vi "ClsDownloadDeviceSpectrumSingleChannelDevice.vi"(8 "error in":errorcluster, 10 "Spectrum Type":i32, 11 "Connection In":u32) -> (0 "error out":errorcluster, 2 "Spectrum":i16[](array[numeric]), 3 "Connection Out":u32)   [LabVIEW 2010]
doc: "Download Device Spectrum:\n\nThis function is used for single channel devices. This function is used for downloading spectrum from first generation CHRocodile devices and CHRocodile 2 devices which have only one measuring channel. For the first generation CHRocodile device the downloaded raw/processed spectrum in confocal mode always has the length of 1024. However different devices can have different valid number of spectrum pixels (less than 1024). These valid pixels reside in the front part of the downloaded spectrum. Sometimes the first a few pixels can also be invalid. Client needs to have a deep look at the spectrum before directly using it. FFT spectrum always has the length of 512, all of which are valid. For CHRocodile2 device, the spectrum length reflects real number of valid pixels.\n\nConnection In[Input]: the connection handle which is initially created by Open Connection subVI.\n\nSpectrum Type[Input]: Spectrum type: 0 for raw spectrum; 1 for processed spectrum in confocal mode; 2 for FFT spectrum in interferometric mode.\n\nSpectrum[Output]: the one dimensional array of requested spectrum.\n\nConnection Out[Output]: the connection handle output which could be used for next subVI refering to the same connection."
uses:
  dependent dlls/CHRocodileDLL.dll
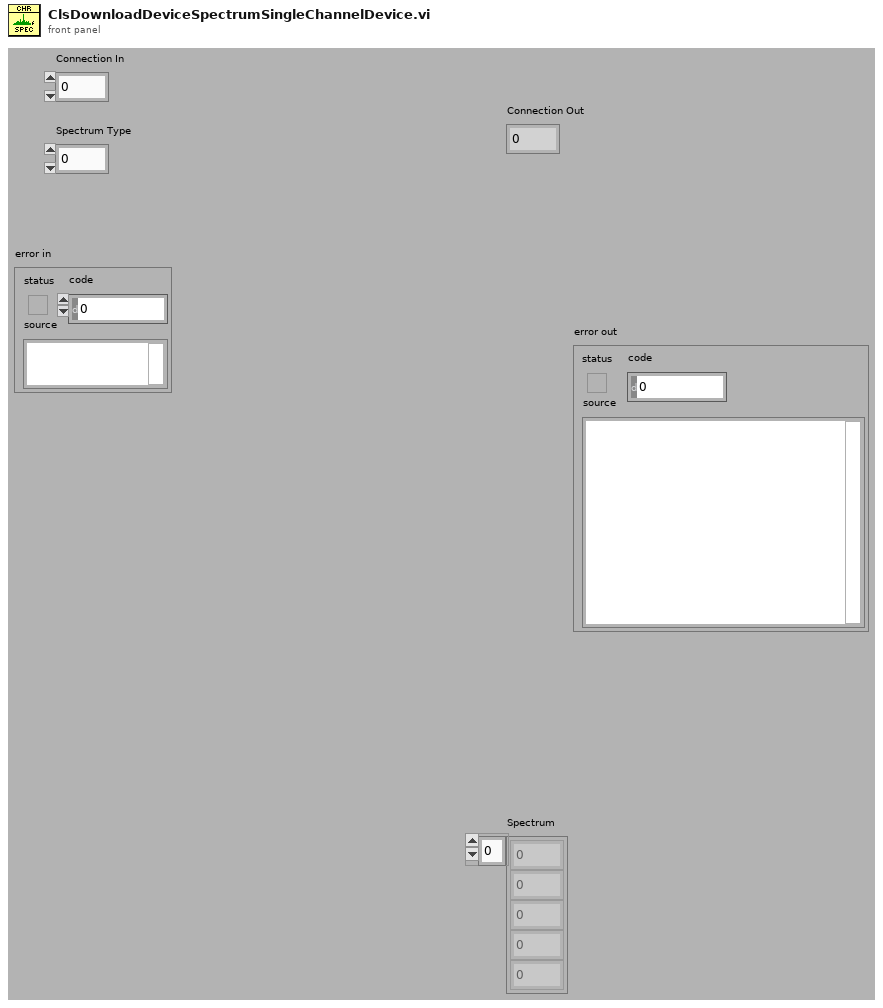
[diagram p1: front panel]
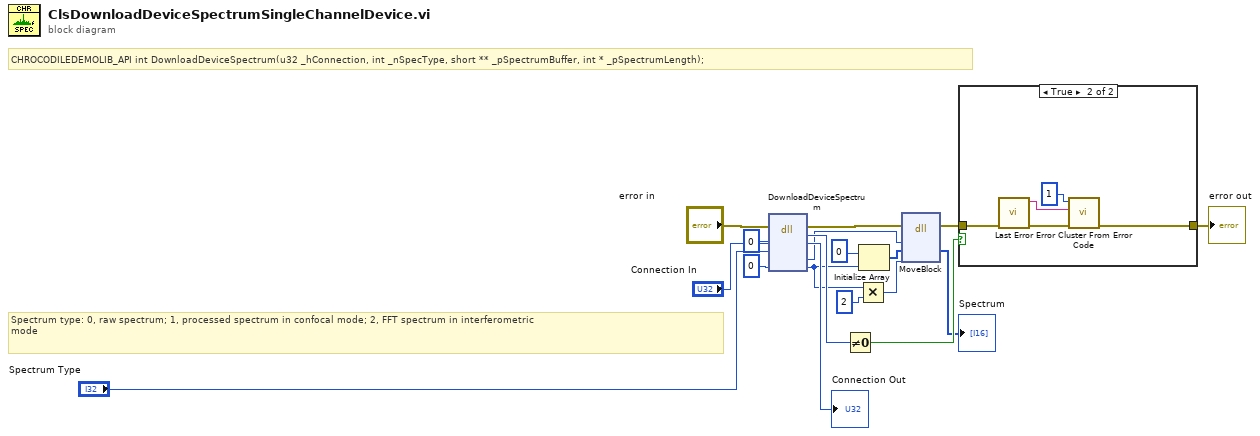
[diagram p0: block diagram]
diagram:
  # "Spectrum type: 0, raw spectrum; 1, processed spectrum in confocal mode; 2, FFT spectrum in interferometric\nmode"
  # "CHROCODILEDEMOLIB_API int DownloadDeviceSpectrum(u32 _hConnection, int _nSpecType, short ** _pSpectrumBuffer, int * _pSpectrumLength);"
  n1 = dll-call lib="C:/Users/y.ji/Desktop/CHRocodile VIs/dependent dlls/CHRocodileDLL.*" fn="DownloadDeviceSpectrum"(error in="error in", "_hConnection"="Connection In", "_nSpecType"="Spectrum Type", "_pSpectrumBuffer"=i64 0, "_pSpectrumLength"=i64 0) -> (error out=w6:errorcluster, "return type"=w13:i32, "_hConnection"=→"Connection Out":u32, "_pSpectrumBuffer"=w4:i64, "_pSpectrumLength"=w3:i64)  [unwired: 3 in, 1 out]
  n2 = Not Equal To 0?(x=w13) -> (x != 0?=w15:bool)
  n3 = Multiply(x=w3, y=2) -> (x*y=w8:i64)
  n4 = Initialize Array(i16 0, w3) -> (w10:i16[])
  n5 = dll-call lib="LabVIEW" fn="MoveBlock"(error in=w6, "Address(pointer)"=w4, "Destination"=w10, "Size"=w8) -> (error out=w5:errorcluster, "Destination"=→"Spectrum":i16[])  [unwired: 5 in, 1 out]
  n6 = case shown="True" w15 {
    tunnel: [w19 w20] -> w14
    tunnel: w5 -> [w19 w23]
    frame False {
    }
    frame True {
      n7 = call "Last Error.vi"("error in (no error)"=w23) -> ("error out"=w22:errorcluster, "Error Message"=w21:string)  [unwired: 9 in]
      n8 = call <vilib>:"Error Cluster From Error Code.vi"("error in (no error)"=w22, "error message (\"\")"=w21, "error code (0)"=1) -> ("error out"=w20:errorcluster)  [unwired: 6 in]
    }
  }
  "error out" <- w14
